vi "LIN_Analyze_signal_values.vi"(10 "ALINData":T2 {"Properties" format="%x"}, 11 "LDF_data_array":T10(array[cluster])) -> (3 "data out":T1)   [LabVIEW 2014]
uses:
  Typedef/TDBProperties.ctl
  Typedef/TDBECUProperties.ctl
  Typedef/TDBFrameProperties.ctl
  Typedef/CAN/TCANSignal.ctl
  Typedef/LIN/TLINSignal.ctl
  Typedef/FlexRay/TFlexRaySignal.ctl
  Typedef/TDBSignalProperties.ctl
  LIN_Function/Typedef/TLibLIN.ctl
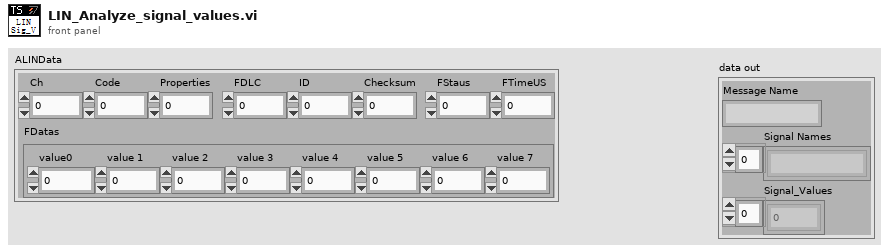
[diagram p1: front panel]
types:
  T1 = cluster{"Message Name":string, "Signal Names":string[], "Signal_Values":dbl[]}
  T2 = typedef "TLibLIN.ctl" = cluster{"Ch":u8, "Code":u8, "Properties":u8, "FDLC":u8, "ID":u8, "Checksum":u8, "FStaus":u8, "FTimeUS":u64, "FDatas":cluster{"value0":u8, "value 1":u8, "value 2":u8, "value 3":u8, "value 4":u8, "value 5":u8, "value 6":u8, "value 7":u8}}
  T3 = typedef "TDBProperties.ctl" = cluster{"FDBIndex":i32, "FSignalCount":i32, "FFrameCount":i32, "FECUCount":i32, "FSupportedChannelMask":u64, "FName":cluster{"数值":u64, "数值 2":u64, "数值 3":u64, "数值 4":u64, "数值 5":u64, "数值 6":u64, "数值 7":u64, "数值 8":u64, "数值 9":u64, "数值 10":u64, "数值 11":u64, "数值 12":u64, "数值 13":u64, "数值 14":u64, "数值 15":u64, "数值 16":u64, "数值 17":u64, "数值 18":u64, "数值 19":u64, "数值 20":u64, "数值 21":u64, "数值 22":u64, "数值 23":u64, "数值 24":u64, "数值 25":u64, "数值 26":u64, "数值 27":u64, "数值 28":u64, "数值 29":u64, "数值 30":u64, "数值 31":u64, "数值 32":u64, "数值 33":u64, "数值 34":u64, "数值 35":u64, "数值 36":u64, "数值 37":u64, "数值 38":u64, "数值 39":u64, "数值 40":u64, "数值 41":u64, "数值 42":u64, "数值 43":u64, "数值 44":u64, "数值 45":u64, "数值 46":u64, "数值 47":u64, "数值 48":u64, "数值 49":u64, "数值 50":u64, "数值 51":u64, "数值 52":u64, "数值 53":u64, "数值 54":u64, "数值 55":u64, "数值 56":u64, "数值 57":u64, "数值 58":u64, "数值 59":u64, "数值 60":u64, "数值 61":u64, "数值 62":u64, "数值 63":u64, "数值 64":u64}, "FComment":cluster{"数值":u64, "数值 2":u64, "数值 3":u64, "数值 4":u64, "数值 5":u64, "数值 6":u64, "数值 7":u64, "数值 8":u64, "数值 9":u64, "数值 10":u64, "数值 11":u64, "数值 12":u64, "数值 13":u64, "数值 14":u64, "数值 15":u64, "数值 16":u64, "数值 17":u64, "数值 18":u64, "数值 19":u64, "数值 20":u64, "数值 21":u64, "数值 22":u64, "数值 23":u64, "数值 24":u64, "数值 25":u64, "数值 26":u64, "数值 27":u64, "数值 28":u64, "数值 29":u64, "数值 30":u64, "数值 31":u64, "数值 32":u64, "数值 33":u64, "数值 34":u64, "数值 35":u64, "数值 36":u64, "数值 37":u64, "数值 38":u64, "数值 39":u64, "数值 40":u64, "数值 41":u64, "数值 42":u64, "数值 43":u64, "数值 44":u64, "数值 45":u64, "数值 46":u64, "数值 47":u64, "数值 48":u64, "数值 49":u64, "数值 50":u64, "数值 51":u64, "数值 52":u64, "数值 53":u64, "数值 54":u64, "数值 55":u64, "数值 56":u64, "数值 57":u64, "数值 58":u64, "数值 59":u64, "数值 60":u64, "数值 61":u64, "数值 62":u64, "数值 63":u64, "数值 64":u64}, "FFlags":u32, "FDBId":u32}
  T4 = typedef "TDBECUProperties.ctl" = cluster{"FDBIndex":i32, "FECUIndex":i32, "FTxFrameCount":i32, "FRxFrameCount":i32, "FName":cluster{"数值":u64, "数值 2":u64, "数值 3":u64, "数值 4":u64, "数值 5":u64, "数值 6":u64, "数值 7":u64, "数值 8":u64, "数值 9":u64, "数值 10":u64, "数值 11":u64, "数值 12":u64, "数值 13":u64, "数值 14":u64, "数值 15":u64, "数值 16":u64, "数值 17":u64, "数值 18":u64, "数值 19":u64, "数值 20":u64, "数值 21":u64, "数值 22":u64, "数值 23":u64, "数值 24":u64, "数值 25":u64, "数值 26":u64, "数值 27":u64, "数值 28":u64, "数值 29":u64, "数值 30":u64, "数值 31":u64, "数值 32":u64, "数值 33":u64, "数值 34":u64, "数值 35":u64, "数值 36":u64, "数值 37":u64, "数值 38":u64, "数值 39":u64, "数值 40":u64, "数值 41":u64, "数值 42":u64, "数值 43":u64, "数值 44":u64, "数值 45":u64, "数值 46":u64, "数值 47":u64, "数值 48":u64, "数值 49":u64, "数值 50":u64, "数值 51":u64, "数值 52":u64, "数值 53":u64, "数值 54":u64, "数值 55":u64, "数值 56":u64, "数值 57":u64, "数值 58":u64, "数值 59":u64, "数值 60":u64, "数值 61":u64, "数值 62":u64, "数值 63":u64, "数值 64":u64}, "FComment":cluster{"数值":u64, "数值 2":u64, "数值 3":u64, "数值 4":u64, "数值 5":u64, "数值 6":u64, "数值 7":u64, "数值 8":u64, "数值 9":u64, "数值 10":u64, "数值 11":u64, "数值 12":u64, "数值 13":u64, "数值 14":u64, "数值 15":u64, "数值 16":u64, "数值 17":u64, "数值 18":u64, "数值 19":u64, "数值 20":u64, "数值 21":u64, "数值 22":u64, "数值 23":u64, "数值 24":u64, "数值 25":u64, "数值 26":u64, "数值 27":u64, "数值 28":u64, "数值 29":u64, "数值 30":u64, "数值 31":u64, "数值 32":u64, "数值 33":u64, "数值 34":u64, "数值 35":u64, "数值 36":u64, "数值 37":u64, "数值 38":u64, "数值 39":u64, "数值 40":u64, "数值 41":u64, "数值 42":u64, "数值 43":u64, "数值 44":u64, "数值 45":u64, "数值 46":u64, "数值 47":u64, "数值 48":u64, "数值 49":u64, "数值 50":u64, "数值 51":u64, "数值 52":u64, "数值 53":u64, "数值 54":u64, "数值 55":u64, "数值 56":u64, "数值 57":u64, "数值 58":u64, "数值 59":u64, "数值 60":u64, "数值 61":u64, "数值 62":u64, "数值 63":u64, "数值 64":u64}}
  T5 = typedef "TDBFrameProperties.ctl" = cluster{"FDBIndex":i32, "FECUIndex":i32, "FFrameIndex":i32, "FIsTx":u8, "FReserved1":u8, "FCycleTimeMs":u16, "TSignalType":i32, "FCANIsDataFrame":u8, "FCANIsStdFrame":u8, "FCANIsEdl":u8, "FCANIsBrs":u8, "FCANIdentifier":i32, "FCANDLC":i32, "FCANDataBytes":i32, "FLINIdentifier":i32, "FLINDLC":i32, "FFRChannelMask":u8, "FFRBaseCycle":u8, "FFRCycleRepetition":u8, "FFRIsStartupFrame":u8, "FFRSlotId":u16, "FFRDLC":u16, "FFRCycleMask":u64, "FSignalCount":i32, "FName":cluster{"数值":u64, "数值 2":u64, "数值 3":u64, "数值 4":u64, "数值 5":u64, "数值 6":u64, "数值 7":u64, "数值 8":u64, "数值 9":u64, "数值 10":u64, "数值 11":u64, "数值 12":u64, "数值 13":u64, "数值 14":u64, "数值 15":u64, "数值 16":u64, "数值 17":u64, "数值 18":u64, "数值 19":u64, "数值 20":u64, "数值 21":u64, "数值 22":u64, "数值 23":u64, "数值 24":u64, "数值 25":u64, "数值 26":u64, "数值 27":u64, "数值 28":u64, "数值 29":u64, "数值 30":u64, "数值 31":u64, "数值 32":u64, "数值 33":u64, "数值 34":u64, "数值 35":u64, "数值 36":u64, "数值 37":u64, "数值 38":u64, "数值 39":u64, "数值 40":u64, "数值 41":u64, "数值 42":u64, "数值 43":u64, "数值 44":u64, "数值 45":u64, "数值 46":u64, "数值 47":u64, "数值 48":u64, "数值 49":u64, "数值 50":u64, "数值 51":u64, "数值 52":u64, "数值 53":u64, "数值 54":u64, "数值 55":u64, "数值 56":u64, "数值 57":u64, "数值 58":u64, "数值 59":u64, "数值 60":u64, "数值 61":u64, "数值 62":u64, "数值 63":u64, "数值 64":u64}, "FComment":cluster{"数值":u64, "数值 2":u64, "数值 3":u64, "数值 4":u64, "数值 5":u64, "数值 6":u64, "数值 7":u64, "数值 8":u64, "数值 9":u64, "数值 10":u64, "数值 11":u64, "数值 12":u64, "数值 13":u64, "数值 14":u64, "数值 15":u64, "数值 16":u64, "数值 17":u64, "数值 18":u64, "数值 19":u64, "数值 20":u64, "数值 21":u64, "数值 22":u64, "数值 23":u64, "数值 24":u64, "数值 25":u64, "数值 26":u64, "数值 27":u64, "数值 28":u64, "数值 29":u64, "数值 30":u64, "数值 31":u64, "数值 32":u64, "数值 33":u64, "数值 34":u64, "数值 35":u64, "数值 36":u64, "数值 37":u64, "数值 38":u64, "数值 39":u64, "数值 40":u64, "数值 41":u64, "数值 42":u64, "数值 43":u64, "数值 44":u64, "数值 45":u64, "数值 46":u64, "数值 47":u64, "数值 48":u64, "数值 49":u64, "数值 50":u64, "数值 51":u64, "数值 52":u64, "数值 53":u64, "数值 54":u64, "数值 55":u64, "数值 56":u64, "数值 57":u64, "数值 58":u64, "数值 59":u64, "数值 60":u64, "数值 61":u64, "数值 62":u64, "数值 63":u64, "数值 64":u64}}
  T6 = typedef "TDBSignalProperties.ctl" = cluster{"FDBIndex":i32, "FECUIndex":i32, "FFrameIndex":i32, "FSignalIndex":i32, "FIsTx":u8, "FReserved1":u8, "FReserved2":u8, "FReserved3":u8, "TSignalType":i32, "TCANSignal":T7, "TLINSignal":T8, "TFlexRaySignal":T9, "FParentFrameId":i32, "FInitValue":dbl, "FName":cluster{"数值":u64, "数值 2":u64, "数值 3":u64, "数值 4":u64, "数值 5":u64, "数值 6":u64, "数值 7":u64, "数值 8":u64, "数值 9":u64, "数值 10":u64, "数值 11":u64, "数值 12":u64, "数值 13":u64, "数值 14":u64, "数值 15":u64, "数值 16":u64, "数值 17":u64, "数值 18":u64, "数值 19":u64, "数值 20":u64, "数值 21":u64, "数值 22":u64, "数值 23":u64, "数值 24":u64, "数值 25":u64, "数值 26":u64, "数值 27":u64, "数值 28":u64, "数值 29":u64, "数值 30":u64, "数值 31":u64, "数值 32":u64, "数值 33":u64, "数值 34":u64, "数值 35":u64, "数值 36":u64, "数值 37":u64, "数值 38":u64, "数值 39":u64, "数值 40":u64, "数值 41":u64, "数值 42":u64, "数值 43":u64, "数值 44":u64, "数值 45":u64, "数值 46":u64, "数值 47":u64, "数值 48":u64, "数值 49":u64, "数值 50":u64, "数值 51":u64, "数值 52":u64, "数值 53":u64, "数值 54":u64, "数值 55":u64, "数值 56":u64, "数值 57":u64, "数值 58":u64, "数值 59":u64, "数值 60":u64, "数值 61":u64, "数值 62":u64, "数值 63":u64, "数值 64":u64}, "FComment":cluster{"数值":u64, "数值 2":u64, "数值 3":u64, "数值 4":u64, "数值 5":u64, "数值 6":u64, "数值 7":u64, "数值 8":u64, "数值 9":u64, "数值 10":u64, "数值 11":u64, "数值 12":u64, "数值 13":u64, "数值 14":u64, "数值 15":u64, "数值 16":u64, "数值 17":u64, "数值 18":u64, "数值 19":u64, "数值 20":u64, "数值 21":u64, "数值 22":u64, "数值 23":u64, "数值 24":u64, "数值 25":u64, "数值 26":u64, "数值 27":u64, "数值 28":u64, "数值 29":u64, "数值 30":u64, "数值 31":u64, "数值 32":u64, "数值 33":u64, "数值 34":u64, "数值 35":u64, "数值 36":u64, "数值 37":u64, "数值 38":u64, "数值 39":u64, "数值 40":u64, "数值 41":u64, "数值 42":u64, "数值 43":u64, "数值 44":u64, "数值 45":u64, "数值 46":u64, "数值 47":u64, "数值 48":u64, "数值 49":u64, "数值 50":u64, "数值 51":u64, "数值 52":u64, "数值 53":u64, "数值 54":u64, "数值 55":u64, "数值 56":u64, "数值 57":u64, "数值 58":u64, "数值 59":u64, "数值 60":u64, "数值 61":u64, "数值 62":u64, "数值 63":u64, "数值 64":u64}}
  T7 = typedef "TCANSignal.ctl" = cluster{"FCANSgnType":u8, "FIsIntel":u8, "FStartBit":i32, "FLength":i32, "FFactor":dbl, "FOffset":dbl}
  T8 = typedef "TLINSignal.ctl" = cluster{"FLINSgnType":u8, "FIsIntel":u8, "FStartBit":i32, "FLength":i32, "FFactor":dbl, "FOffset":dbl}
  T9 = typedef "TFlexRaySignal.ctl" = cluster{"FFRSgnType":u8, "FCompuMethod":u8, "FReserved":u8, "FIsIntel":u8, "FStartBit":i32, "FUpdateBit":i32, "FLength":i32, "FFactor":dbl, "FOffset":dbl, "FActualStartBit":i32, "FActualUpdateBit":i32}
  T10 = cluster{"db_properties":T3, "ECU_array":cluster{"TDBECUProperties":T4, "TX_Frame_array":cluster{"Frame_Properties":T5, "signal_array":T6[]}[], "RX_Frame_array":cluster{"Frame_Properties":T5, "signal_array":T6[]}[]}[]}[]
  T11 = cluster{"TDBECUProperties":T4, "TX_Frame_array":cluster{"Frame_Properties":T5, "signal_array":T6[]}[], "RX_Frame_array":cluster{"Frame_Properties":T5, "signal_array":T6[]}[]}[]
  T12 = cluster{"Frame_Properties":T5, "signal_array":T6[]}[]
  T13 = cluster{"value0":u8, "value 1":u8, "value 2":u8, "value 3":u8, "value 4":u8, "value 5":u8, "value 6":u8, "value 7":u8}
  T14 = cluster{"数值":u64, "数值 2":u64, "数值 3":u64, "数值 4":u64, "数值 5":u64, "数值 6":u64, "数值 7":u64, "数值 8":u64, "数值 9":u64, "数值 10":u64, "数值 11":u64, "数值 12":u64, "数值 13":u64, "数值 14":u64, "数值 15":u64, "数值 16":u64, "数值 17":u64, "数值 18":u64, "数值 19":u64, "数值 20":u64, "数值 21":u64, "数值 22":u64, "数值 23":u64, "数值 24":u64, "数值 25":u64, "数值 26":u64, "数值 27":u64, "数值 28":u64, "数值 29":u64, "数值 30":u64, "数值 31":u64, "数值 32":u64, "数值 33":u64, "数值 34":u64, "数值 35":u64, "数值 36":u64, "数值 37":u64, "数值 38":u64, "数值 39":u64, "数值 40":u64, "数值 41":u64, "数值 42":u64, "数值 43":u64, "数值 44":u64, "数值 45":u64, "数值 46":u64, "数值 47":u64, "数值 48":u64, "数值 49":u64, "数值 50":u64, "数值 51":u64, "数值 52":u64, "数值 53":u64, "数值 54":u64, "数值 55":u64, "数值 56":u64, "数值 57":u64, "数值 58":u64, "数值 59":u64, "数值 60":u64, "数值 61":u64, "数值 62":u64, "数值 63":u64, "数值 64":u64}
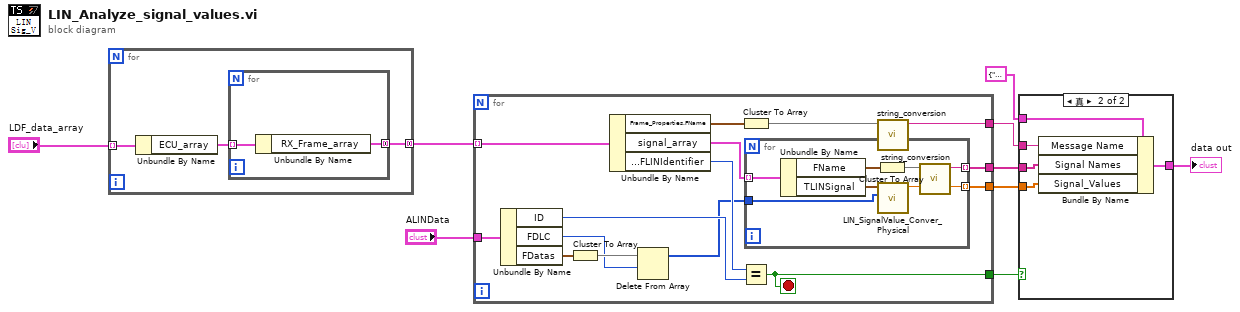
[diagram p0: block diagram]
diagram:
  n1 = for {
    tunnel: "LDF_data_array" -> [w12] mode=indexing
    tunnel: [w10] -> w8 mode=concatenating
    n2 = Unbundle By Name(w12) -> ("ECU_array"=w11:T11)
    n3 = for {
      tunnel: w11 -> [w14] mode=indexing
      tunnel: [w13] -> w10 mode=concatenating
      n4 = Unbundle By Name(w14) -> ("RX_Frame_array"=w13:T12)
    }
  }
  n5 = for {
    tunnel: w8 -> [w29] mode=indexing
    tunnel: "ALINData" -> [w25]
    tunnel: [w22] -> w6
    tunnel: [w21] -> w5
    tunnel: [w17] -> w4
    tunnel: [w15] -> w1
    stop <- w15 stop-if-true
    n6 = Unbundle By Name(w25) -> ("ID"=w24:u8, "FDLC"=w18:u8, "FDatas"=w20:T13)
    n7 = Cluster To Array(cluster=w20) -> (array=w19:u8[])
    n8 = Unbundle By Name(w29) -> ("Frame_Properties.FName"=w27:T14, "signal_array"=w26:T6[], "Frame_Properties.FLINIdentifier"=w23:i32)
    n9 = Delete From Array(array=w19, length=w18) -> (array with subset deleted=w16:u8[])  [unwired: 1 in, 1 out]
    n10 = Cluster To Array(cluster=w27) -> (array=w28:u64[])
    n11 = Equal?(x=w23, y=w24) -> (x = y?=w15:bool)
    n12 = for {
      tunnel: w26 -> [w36] mode=indexing
      tunnel: [w32] -> w21 mode=indexing
      tunnel: w16 -> [w31]
      tunnel: [w30] -> w17 mode=indexing
      n13 = Unbundle By Name(w36) -> ("FName"=w35:T14, "TLINSignal"=w33:T8)
      n14 = Cluster To Array(cluster=w35) -> (array=w34:u64[])
      n15 = call "LIN_SignalValue_Conver_Physical.vi"("FDatas"=w31, "TLINSignal"=w33) -> ("Signal Value"=w30:dbl)  [unwired: 9 in]
      n16 = call "string_conversion.vi"("FName"=w34) -> ("string"=w32:string)  [unwired: 10 in]
    }
    n17 = call "string_conversion.vi"("FName"=w28) -> ("string"=w22:string)  [unwired: 10 in]
  }
  n18 = case shown="真" w1 {
    tunnel: w6 -> [_ w42]
    tunnel: w5 -> [_ w41]
    tunnel: w4 -> [_ w40]
    tunnel: [w37 w39] -> w3
    tunnel: T1 {"Message Name"="", "Signal Names"=[], "Signal_Values"=[]} ("data out") -> [w37 w38]
    frame False {
    }
    frame True {
      n19 = Bundle By Name(cluster=w38, "Message Name"=w42, "Signal Names"=w41, "Signal_Values"=w40) -> (w39:T1)
    }
  }
  "data out" <- w3
